vi "Connect.vi"(8 "error in (no error)":errorcluster, 11 "FW Arduino Control in":refnum<class "FW Arduino Control.lvclass">) -> (0 "error out":errorcluster, 3 "FW Arduino Control out":refnum<class "FW Arduino Control.lvclass">)   [LabVIEW 2022 SP3, in "FW Arduino Control.lvclass"]
uses:
  FW Arduino Control.lvclass
  C:/Development/rimas/RIMAS/Filter Wheel/Filter Wheel Object/Filter Wheel.lvclass
  Filter Wheel Object/Filter Wheel.lvclass/Filter Wheel.ctl
  FW Arduino Control.lvclass/FW Arduino Control.ctl
  86b5e62a-99a7-4932-a2e6-7eaa98965210.vi
  Filter Wheel Object/Read Homing 2.vi
  <vilib>/Instr/_visa.llb/VISA Configure Serial Port (Instr).vi
  Filter Wheel Object/Filter Wheel.lvclass
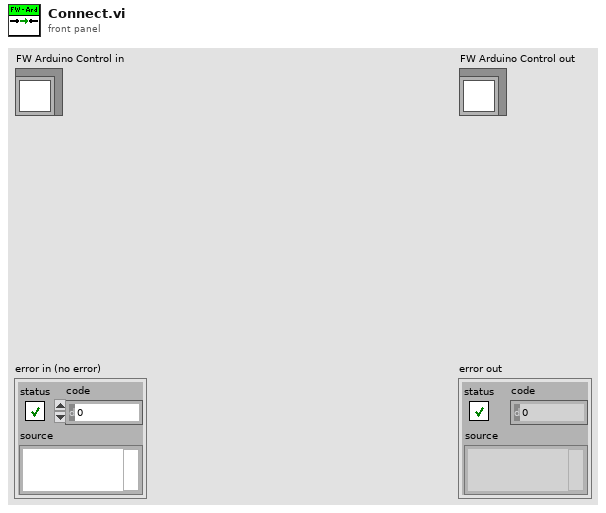
[diagram p1: front panel]
types:
  T1 = typedef "Filter Wheel Arduino Homing cluster.ctl" = cluster{"Direction (F: CW)":bool, "Speed":i32, "Accel":i32, "Error Cnts":i32, "Homing Delta":i32}
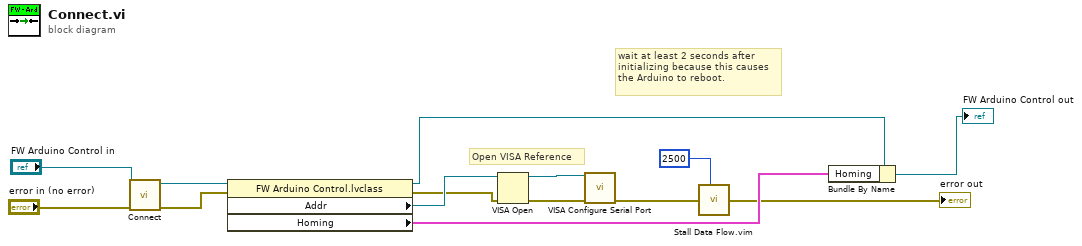
[diagram p0: block diagram]
diagram:
  # "wait at least 2 seconds after initializing because this causes the Arduino to reboot."
  # "Open VISA Reference"
  n1 = call-parent "Connect.vi"("error in (no error)"="error in (no error)", "Filter Wheel in"="FW Arduino Control in") -> ("error out"=w3:errorcluster, "Filter Wheel out"=w6:refnum<class "FW Arduino Control.lvclass">)  [unwired: 8 in]
  n2 = property class="FW Arduino Control.lvclass"(reference=w6, error in=w3) -> (reference out=w5:refnum<class "FW Arduino Control.lvclass">, error out=w11:errorcluster, "Addr"=w12:refnum<visa-resource-name>, "Homing"=w2:T1[])
  n3 = VISA Open(error in (no error)=w11, VISA resource name=w12) -> (VISA resource name=w10:refnum<visa-resource-name>, error out=w9:errorcluster)  [unwired: 3 in]
  n4 = call-poly "VISA Configure Serial Port"("VISA resource name"=w10, "error in (no error)"=w9) -> ("error out"=w8:errorcluster)  [unwired: 12 in, 1 out]
  n5 = call "Stall Data Flow.vim"("value in"=w8, "milliseconds to wait"=u32 2500) -> ("value out"=→"error out":errorcluster)  [unwired: 1 out]
  n6 = Bundle By Name(cluster=w5, "Homing"=w2) -> (→"FW Arduino Control out":refnum<class "FW Arduino Control.lvclass">)
